vi "Load Service.vi"(8 "error in (no error)":errorcluster, 9 "Database path":path, 10 "Paquete":string, 11 "Manejo Turnos in":refnum<class "Manejo Turnos.lvclass">) -> (0 "error out":errorcluster, 3 "Manejo Turnos out":refnum<class "Manejo Turnos.lvclass">)   [LabVIEW 2020, in "Manejo Turnos.lvlib" / "Manejo Turnos.lvclass"]
uses:
  Manejo Turnos.lvclass
  C:/Program Files (x86)/National Instruments/LabVIEW 2020/vi.lib/ActorFramework/Actor/Actor.lvclass
  Manejo Turnos.lvclass/Manejo Turnos.ctl
  <vilib>/ActorFramework/Actor/Actor.lvclass/Actor.ctl
  <vilib>/ActorFramework/Message Enqueuer/Message Enqueuer.lvclass/Message Enqueuer.ctl
  <vilib>/drjdpowell/SQLite Library/SQL Connection/Open (path).vi
  <vilib>/ActorFramework/Message Enqueuer/Init from Existing Queue.vi
  <vilib>/ActorFramework/Message Enqueuer/Enqueue.vi
  <vilib>/drjdpowell/SQLite Library/SQL Connection/Open (string).vi
  Manejo Turnos Messages/Read Service Msg/Read Service Msg.lvclass
  C:/Program Files (x86)/National Instruments/LabVIEW 2020/vi.lib/ActorFramework/Message/Message.lvclass
  <vilib>/AdvancedString/Path To Command Line String.vi
  <vilib>/ActorFramework/Message Priority Queue/Priority Enqueue.vi
  <vilib>/drjdpowell/SQLite Library/SQL Connection/Execute SQL (No results).vi
  <vilib>/drjdpowell/SQLite Library/SQL Connection/Connection.lvclass
  <vilib>/ActorFramework/Message Enqueuer/Message Enqueuer.lvclass
  <vilib>/drjdpowell/SQLite Library/SQLite.lvlib
  <vilib>/ActorFramework/Actor/Actor.lvclass
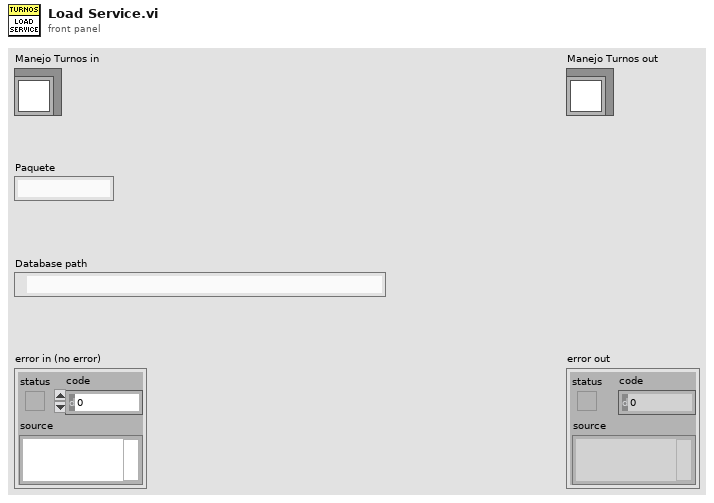
[diagram p1: front panel]
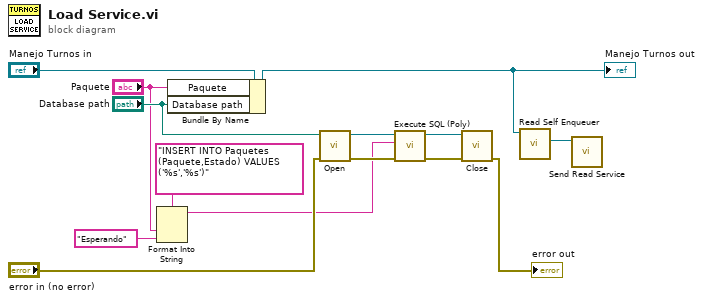
[diagram p0: block diagram]
diagram:
  n1 = Format Into String(format string="INSERT INTO Paquetes (Paquete,Estado) VALUES ('%s','%s')", "Paquete", "Esperando" ("Service Status")) -> (resulting string=w4:string)  [unwired: 2 in, 1 out]
  n2 = Bundle By Name(cluster="Manejo Turnos in", "Paquete"="Paquete", "Database path"="Database path") -> (w2:refnum<class "Manejo Turnos.lvclass">)
  "Manejo Turnos out" <- w2
  n3 = call-poly <vilib>:"Open.vi"("error in (no error)"="error in (no error)", "db file"="Database path") -> ("error out"=w12:errorcluster, "SQLite Connection"=w9:refnum<class "Connection.lvclass">)  [unwired: 8 in]
  n4 = call-poly <vilib>:"Execute SQL (Poly).vi"("error in (no error)"=w12, "SQL"=w4, "SQLite Connection in"=w9) -> ("error out"=w13:errorcluster, "SQLite Connection"=w8:refnum<class "Connection.lvclass">)  [unwired: 7 in]
  n5 = call-dynamic "Close.vi"("error in (no error)"=w13, "SQLite Connection in"=w8) -> ("error out"=→"error out":errorcluster)  [unwired: 9 in]
  n6 = call <vilib>:"Read Self Enqueuer.vi"("Actor"=w2) -> ("Self Enqueuer"=w1:refnum<class "Message Enqueuer.lvclass">)  [unwired: 10 in]
  n7 = call "Send Read Service.vi"("Message Enqueuer"=w1) -> ()  [unwired: 9 in, 2 out]
